vi "Bounce Window_User Accounts_Data.vi"(7 "Table_Action":T5, 8 "Error in":errorcluster, 9 "Row":i32, 10 "Data Array In":T1[](array[typedef]), 11 "User Account Data In":T1={"帳號 :"="", "權限等級："=enum."開發人員", "建立時間："="", "修改時間："="", "到期時間："="", "狀態："=enum."可使用", "期限："=enum."一天", "密碼："=""}) -> (0 "Error Out":errorcluster, 2 "User Account Data Out":T1={"帳號 :"="", "權限等級："=enum."開發人員", "建立時間："="", "修改時間："="", "到期時間："="", "狀態："=enum."可使用", "期限："=enum."一天", "密碼："=""}, 3 "Data Array Out":T1[](array[typedef]))   [LabVIEW 2015]
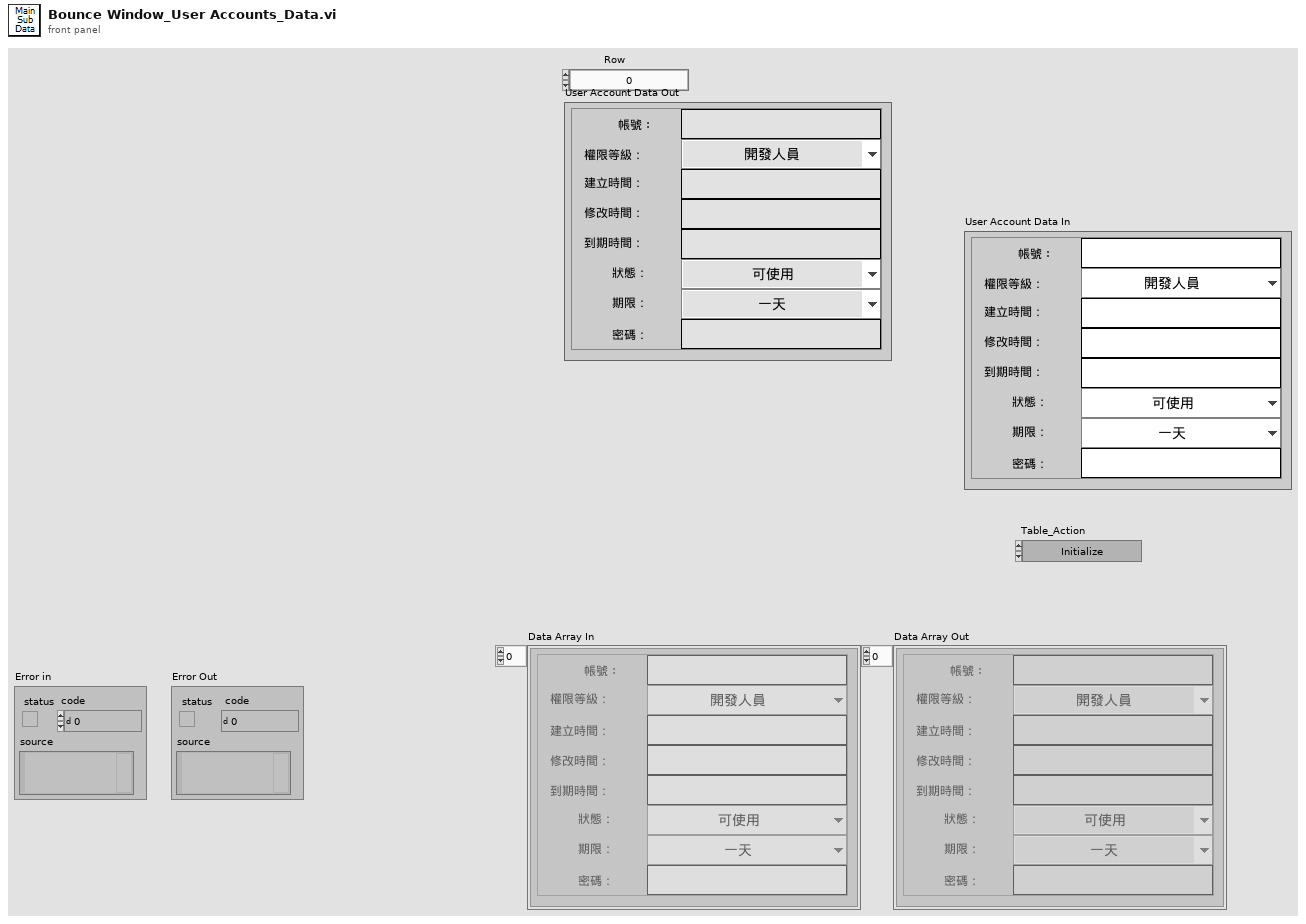
[diagram p1: front panel]
types:
  T1 = typedef "Control_User account_Data.ctl" = cluster{"帳號 :":string, "權限等級：":T2, "建立時間：":string, "修改時間：":string, "到期時間：":string, "狀態：":T3, "期限：":T4, "密碼：":string}
  T2 = typedef "Control_User account_Permissions.ctl" = enum16{"開發人員", "管理者", "工程師", "作業員"}
  T3 = typedef "Control_User Accounts_Status.ctl" = enum16{"可使用", "不可使用"}
  T4 = typedef "Control_User account_Date.ctl" = enum16{"零天", "一天", "七天", "一個月", "一年", "三年"}
  T5 = typedef "Control_Bounce Window_User Accounts_Data Action" = enum16{"Initialize", "Set Data", "Set Data Array", "Replace Data", "Delete Data", "Get Data", "Get Data Array"}
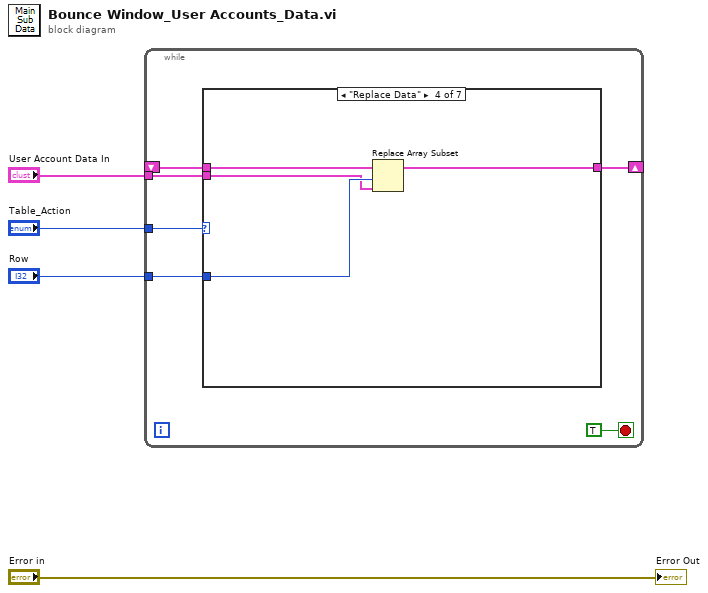
[diagram p0: block diagram]
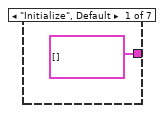
[diagram p2: hidden frame]
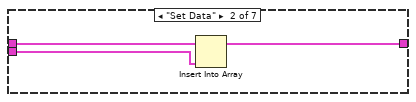
[diagram p3: hidden frame]
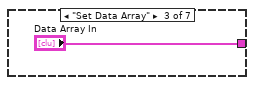
[diagram p4: hidden frame]
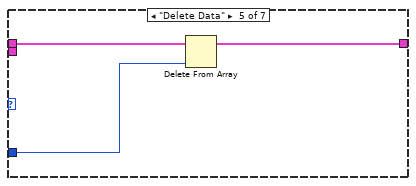
[diagram p5: hidden frame]
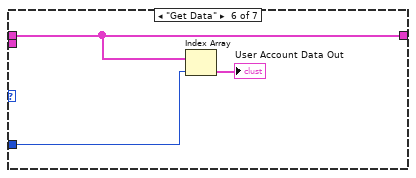
[diagram p6: hidden frame]
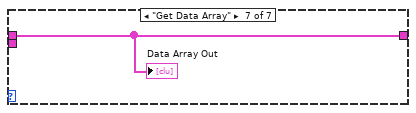
[diagram p7: hidden frame]
diagram:
  n1 = while {
    tunnel: "Table_Action" -> [w9]
    tunnel: "User Account Data In" -> [w8]
    shift-right: [w7] -> _
    shift-left: _ -> [w6]
    tunnel: "Row" -> [w5]
    stop <- TRUE stop-if-true
    n2 = case shown="\"Replace Data\"" w9 {
      tunnel: w8 -> [_ w12 _ w16 _ _ _]
      tunnel: [T1[] [] w13 "Data Array In" w18 w21 w24 w26] -> w7
      tunnel: w6 -> [_ w14 _ w19 w22 w24 w26]
      tunnel: w5 -> [_ _ _ w17 w20 w25 _]
      frame "Initialize", Default {
      }
      frame "Set Data" {
        n3 = Insert Into Array(array=w14, new element=w12) -> (w13:T1[])  [unwired: 1 in]
      }
      frame "Set Data Array" {
      }
      frame "Replace Data" {
        n4 = Replace Array Subset(array=w19, new element=w16, index=w17) -> (w18:T1[])
      }
      frame "Delete Data" {
        n5 = Delete From Array(array=w22, index=w20) -> (array with subset deleted=w21:T1[])  [unwired: 1 in, 1 out]
      }
      frame "Get Data" {
        n6 = Index Array(array=w24, index=w25) -> (element=→"User Account Data Out":T1)
      }
      frame "Get Data Array" {
        "Data Array Out" <- w26
      }
    }
  }
  "Error Out" <- "Error in"
